vi "Set Bucket RequestPayment Configuration.vi"(7 "RequestPayment Configuration":T1, 8 "error in (no error)":errorcluster, 9 "Bucket":string) -> (0 "error out":errorcluster)   [LabVIEW 2011, in "LV Interface for Amazon S3.lvlib"]
doc: "This operation <B>sets the RequestPayment configuration</B> of a bucket. By default, <B>the bucket owner pays for downloads from the bucket</B>. This configuration parameter enables the bucket owner (only) to specify that the person requesting the download will be charged for the download."
uses:
  LV Interface for Amazon S3.lvlib
  Typedefs/AMZ_S3_API_RequestPaymentConfig.ctl
  Typedefs/AMZ_S3_Payer.ctl
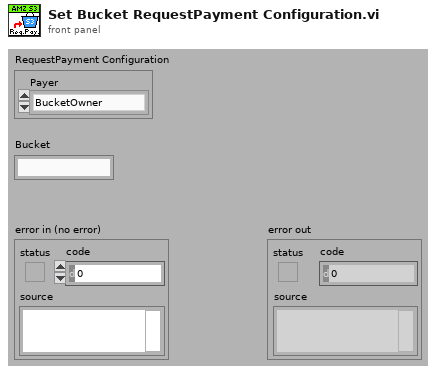
[diagram p1: front panel]
types:
  T1 = typedef "LV Interface for Amazon S3.lvlib/AMZ_S3_API_RequestPaymentConfig.ctl" = cluster{"Payer":T2}
  T2 = typedef "LV Interface for Amazon S3.lvlib/AMZ_S3_Payer.ctl" = enum16{"BucketOwner", "Requester"}
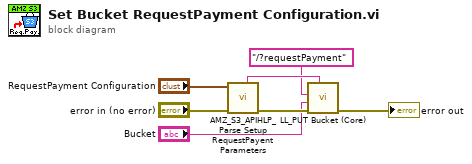
[diagram p0: block diagram]
diagram:
  n1 = call "AMZ_S3_APIHLP_Parse Setup RequestPayent Parameters.vi"("error in (no error)"="error in (no error)", "RequestPaymentConfiguration"="RequestPayment Configuration") -> ("error out"=w5:errorcluster, "PUT Data"=w4:string)  [unwired: 8 in]
  n2 = call "LL_PUT Bucket (Core).vi"("Data"=w4, "error in (no error)"=w5, "Bucket"="Bucket", "Path and query string"="/?requestPayment") -> ("error out"=→"error out":errorcluster)  [unwired: 4 in, 3 out]
